vi "Strain Gauge Motion [FPGA Main].vi"() -> ()   [LabVIEW 2017]
doc: "Use this VI to control the cRIO Demo Kit motor and motor drive with a simple set of commands. You can operate the drive in 2 different modes. By default, you can input a velocity setpoint withing +20 or -20 rotations per second and the motor will move to that velocity, limited by the maximum acceleration input. Alternatively, you can turn on the heater mode. This will use the motor like a heater coil within the demo kit by setting the velocity to zero, but enabling full holding current through the drive. You can use the thermocouple in the demo kit to read the temperature of the motor windings. Turn the heating coil on and off by enabling and disabling the drive.\n\nUSING THIS VI: You can run this VI as the top level VI for an easy motion or heater component. Or you can modify this VI to run as a component of a main FPGA application. To do this, replace the front panel objects with target scoped registers, UDVs, or global variables."
uses:
  <vilib>/Platform/TimedLoop/XDataNode/timing_clust.ctl
  <vilib>/Platform/TimedLoop/XDataNode/nitl_modes.ctl
  <vilib>/Platform/TimedLoop/XDataNode/wakeup.ctl
  <vilib>/LabVIEW Targets/FPGA/cRIO/shared/nicrio_ModuleControls/nicrio_cRIO-9503_DriveStatus.ctl
  <vilib>/Motion/MotorControl/_s/nism.stepper.currentScheduler.config.ctl
  <vilib>/Motion/MotorControl/_s/nism.microstepping.rate.ctl
  <vilib>/Motion/MotorControl/_s/nism.pi.gains.sgl.ctl
  <vilib>/Motion/MotorControl/_s/nism.pi.c.currentFeedback.sgl.ctl
  <vilib>/Motion/MotorControl/_s/nism.mdo.antiResonanceData.ctl
  <vilib>/Motion/MotorControl/_s/nism.stepper.currentScheduler.torqueSmoothingCoefficients.ctl
  <vilib>/Motion/MotorControl/_s/nism.pwm.outputs.4phase.ctl
  <vilib>/rvi/DataTransferAndStorage/Container/Common/niFpgaContainerGetUniqueNameForEmu.vi
  <vilib>/rvi/DataTransferAndStorage/Container/Common/niFpgaContainerSetEmuInfo.vi
  <vilib>/rvi/eio/common/nirviEmuReportErrorAndStop.vi
  <vilib>/rvi/Emulation/niFpgaGetClockAttributes.vi
  <vilib>/rvi/Emulation/niFpgaSctlEmulationGetInTimedLoop.vi
  <vilib>/rvi/Emulation/niFpgaEmulationReportErrorSimple.vi
  <vilib>/rvi/eio/common/nirviEmuTemplateMethod_errors.vi
  <vilib>/rvi/Emulation/niFpgaEmulationIsFPGAContextNoSignature.vi
  <vilib>/rvi/Memory/Memory_Emulation/niFpgaMemoryEmulationCacheClearOnFirstRun.vi
  <vilib>/rvi/Memory/Memory_Emulation/nirvimemoryEmulationManagerCache_MakeExclusive.vi
  <vilib>/rvi/Memory/Memory_Emulation/niFpgaMemoryEmulationValidateCache.vi
  <vilib>/rvi/Memory/Memory_Emulation/nirvimemoryEmulationManagerCache_InsertValue.vi
  <vilib>/Utility/error.llb/Clear Errors.vi
  <vilib>/rvi/Memory/Memory_Emulation/nirvimemoryEmulationManagerCache_ReleaseExclusive.vi
  <vilib>/rvi/Memory/Memory_Emulation/nirvimemoryEmulationManagerCache_GetValue.vi
  <vilib>/rvi/Memory/Memory_Emulation/nirvimemoryEmulationManagerCache_SetValue.vi
  <vilib>/rvi/Emulation/niFpgaProcessEmulError.vi
  <vilib>/rvi/Emulation/niFpgaCriticalErrorInLSC.vi
  <vilib>/rvi/occurrence/nirviWaitOnOccurrenceBase.vi
  <vilib>/Motion/MotorControl/_s/nism.rateLimiter.v.fxp.vi
  <vilib>/Motion/MotorControl/_s/nism.stepResolver.fxp.64.32.vi
  <vilib>/Motion/MotorControl/_s/nism.stepper.currentScheduler.advanced.single.vi
  <vilib>/Motion/MotorControl/_s/nism.pi.c.sgl.2phase.2.noAW.vi
  <vilib>/Motion/MotorControl/_s/nism.antiResonance.single.vi
  <vilib>/Motion/MotorControl/_s/nism.9503VoltageTransform.fxp.vi
  <vilib>/rvi/LocalResourceManager/LocalResourceManager.xnode
  <vilib>/eio/EIOMethodNode/EIOMethodNode.xnode
  <vilib>/rvi/DataTransferAndStorage/Container/XNode/niFpgaContainer.xnode
  <vilib>/rvi/DataTransferAndStorage/Register/Emulation/niFpgaRegisterEmulation.vi
  <vilib>/Platform/TimedLoop/XDataNode/XDataNode.xnode
  <vilib>/eio/EIONode/EIONode.xnode
  <vilib>/Motion/MotorControl/NI_SoftMotion_MotorControlIP.lvlib
  <vilib>/Platform/TimedLoop/XDataNode/XDNodeRunTimeDep.lvlib
  <vilib>/Motion/MotorControl/_s/nism.incremental.indexCriteria.ctl
  <vilib>/Motion/MotorControl/_s/nism.encoder.incremental.config.ctl
  <vilib>/Motion/MotorControl/_s/nism.incremental.p.2.vi
panel:
  out "Strain Gauge":sgl
  in  "Heater Mode":bool
  in  "Velocity Setpoint (rev/sec)":sgl caption="velocity setpoint"
  in  "Maximum Acceleration":T1(ring)=enum."High"
  out "Control Loop Timer":u32
  out "Anti-Resonance Enabled?":bool
  out "Pulse Per Revolution":bool
  out "Velocity (rev/sec)":fxp<+/-,32,16> caption="xi" format="%.41g"
  in  "Clear Faults":bool
  in  "Enable Drive":bool
  out "Module Fault Code":u16
  out "Module Fault?":bool
  # "Velocity is limited to +10 or -10 revolutions per second. Positive velocity setpoints equate to counter clockwise rotation.\n\nMax acceleration choices limit the rate of acceleration when changing velocity setpoints.\n\nHeater Mode will stop the motor and always keep full current through the motor windings, generating more heat.\n\nVelocity is the measured encoder velocity and works without the drive enabled. Pulse Per Revolution is the Z encoder pulse and occors exactly once for each revolution."
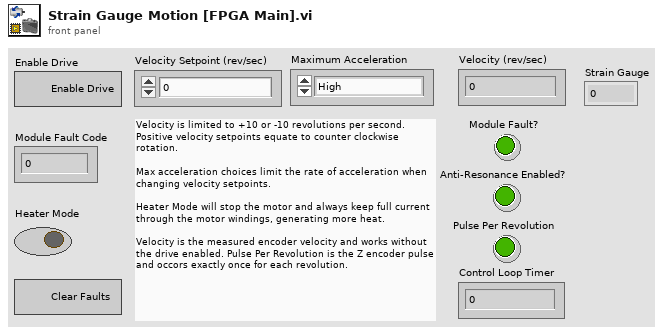
[diagram p1: front panel]
types:
  T1 = enum8{"Extremely Low", "Very Low", "Low", "Medium", "High", "Highest"}
  T2 = typedef "NI_SoftMotion_MotorControlIP.lvlib/nism.encoder.incremental.config.ctl" = cluster{"line a active high?":bool, "line b active high?":bool, "index active high?":bool}
  T3 = typedef "NI_SoftMotion_MotorControlIP.lvlib/nism.incremental.indexCriteria.ctl" = cluster{"a":bool, "b":bool, "z":bool}
  T4 = typedef "XDNodeRunTimeDep.lvlib/timing_clust.ctl" = cluster{"Expected End [f-1]":u64, "Actual End [f-1]":u64, "Finished Late? [f-1]":bool, "Expected End [i-1]":u64, "Actual End [i-1]":u64, "Finished Late? [i-1]":bool, "Expected Start [i]":u64, "Actual Start [i]":u64, "Expected Start [f]":u64, "Actual Start [f]":u64, "Source Name":string, "Structure Name":string, "Period":i64, "Deadline":i64, "Offset":i64, "Start":i64, "Priority":i32, "Timeout":i32, "Mode":T5, "Wakeup Reason":T6, "Error":errorcluster, "Source Type":string, "Secondary Source Type":string, "Global End Time":u64, "Global Start Time":u64, "Frame Duration":u64, "Iteration Duration":u64, "Assigned CPU":i32, "I/O Scan Engine Mode":u32}
  T5 = typedef "XDNodeRunTimeDep.lvlib/nitl_modes.ctl" = enum32{"No Change", "Process missed periods, maintain original phase", "Discard missed periods, maintain original phase", "Process missed periods, ignore original phase", "Discard missed periods, ignore original phase"}
  T6 = typedef "XDNodeRunTimeDep.lvlib/wakeup.ctl" = enum32{"Normal", "Aborted", "Asynchronous wakeup", "Timing source error", "Timed loop error", "Timeout"}
  T7 = typedef "nicrio_cRIO-9503_DriveStatus.ctl" = enum8{"Drive Disabled (Disabled by fault)", "Drive Disabled (Disabled by software)", "Drive Enabled"}
  T8 = typedef "NI_SoftMotion_MotorControlIP.lvlib/nism.pwm.outputs.4phase.ctl" = cluster{"a+":fxp<+/-,16,1>, "a-":fxp<+/-,16,1>, "b+":fxp<+/-,16,1>, "b-":fxp<+/-,16,1>}
  T9 = typedef "NI_SoftMotion_MotorControlIP.lvlib/nism.stepper.currentScheduler.torqueSmoothingCoefficients.ctl" = cluster{"current scheduler : torque smoothing : torque smoothing gain":sgl, "torque smoothing phase":fxp<+/-,16,1>}
  T10 = typedef "NI_SoftMotion_MotorControlIP.lvlib/nism.mdo.antiResonanceData.ctl" = cluster{"coefficient 0":sgl, "coefficient 1":sgl, "coefficient 2":sgl, "coefficient 3":sgl, "coefficient 4":sgl, "coefficient 5":sgl}
  T11 = typedef "NI_SoftMotion_MotorControlIP.lvlib/nism.pi.c.currentFeedback.sgl.ctl" = cluster{"phase a":sgl, "phase b":sgl}
  T12 = typedef "NI_SoftMotion_MotorControlIP.lvlib/nism.pi.gains.sgl.ctl" = cluster{"kp":sgl, "ki":sgl}
  T13 = typedef "NI_SoftMotion_MotorControlIP.lvlib/nism.microstepping.rate.ctl" = enum8{"1 (Full Step)", "2 (Half Step)", "4", "8", "16", "32", "64", "128", "256"}
  T14 = typedef "NI_SoftMotion_MotorControlIP.lvlib/nism.stepper.currentScheduler.config.ctl" = cluster{"rated phase current":sgl, "phase current offset(a)":sgl, "phase current offset(b)":sgl, "reduced current":sgl, "curr. reduction del.":u16}
  T15 = typedef "NI_SoftMotion_MotorControlIP.lvlib/nism.pi.c.currentSetpoint.sgl.ctl" = cluster{"phase a":sgl, "phase b":sgl}
  T16 = typedef "NI_SoftMotion_MotorControlIP.lvlib/nism.pi.c.voltage.sgl.ctl" = cluster{"phase a":sgl, "phase b":sgl}
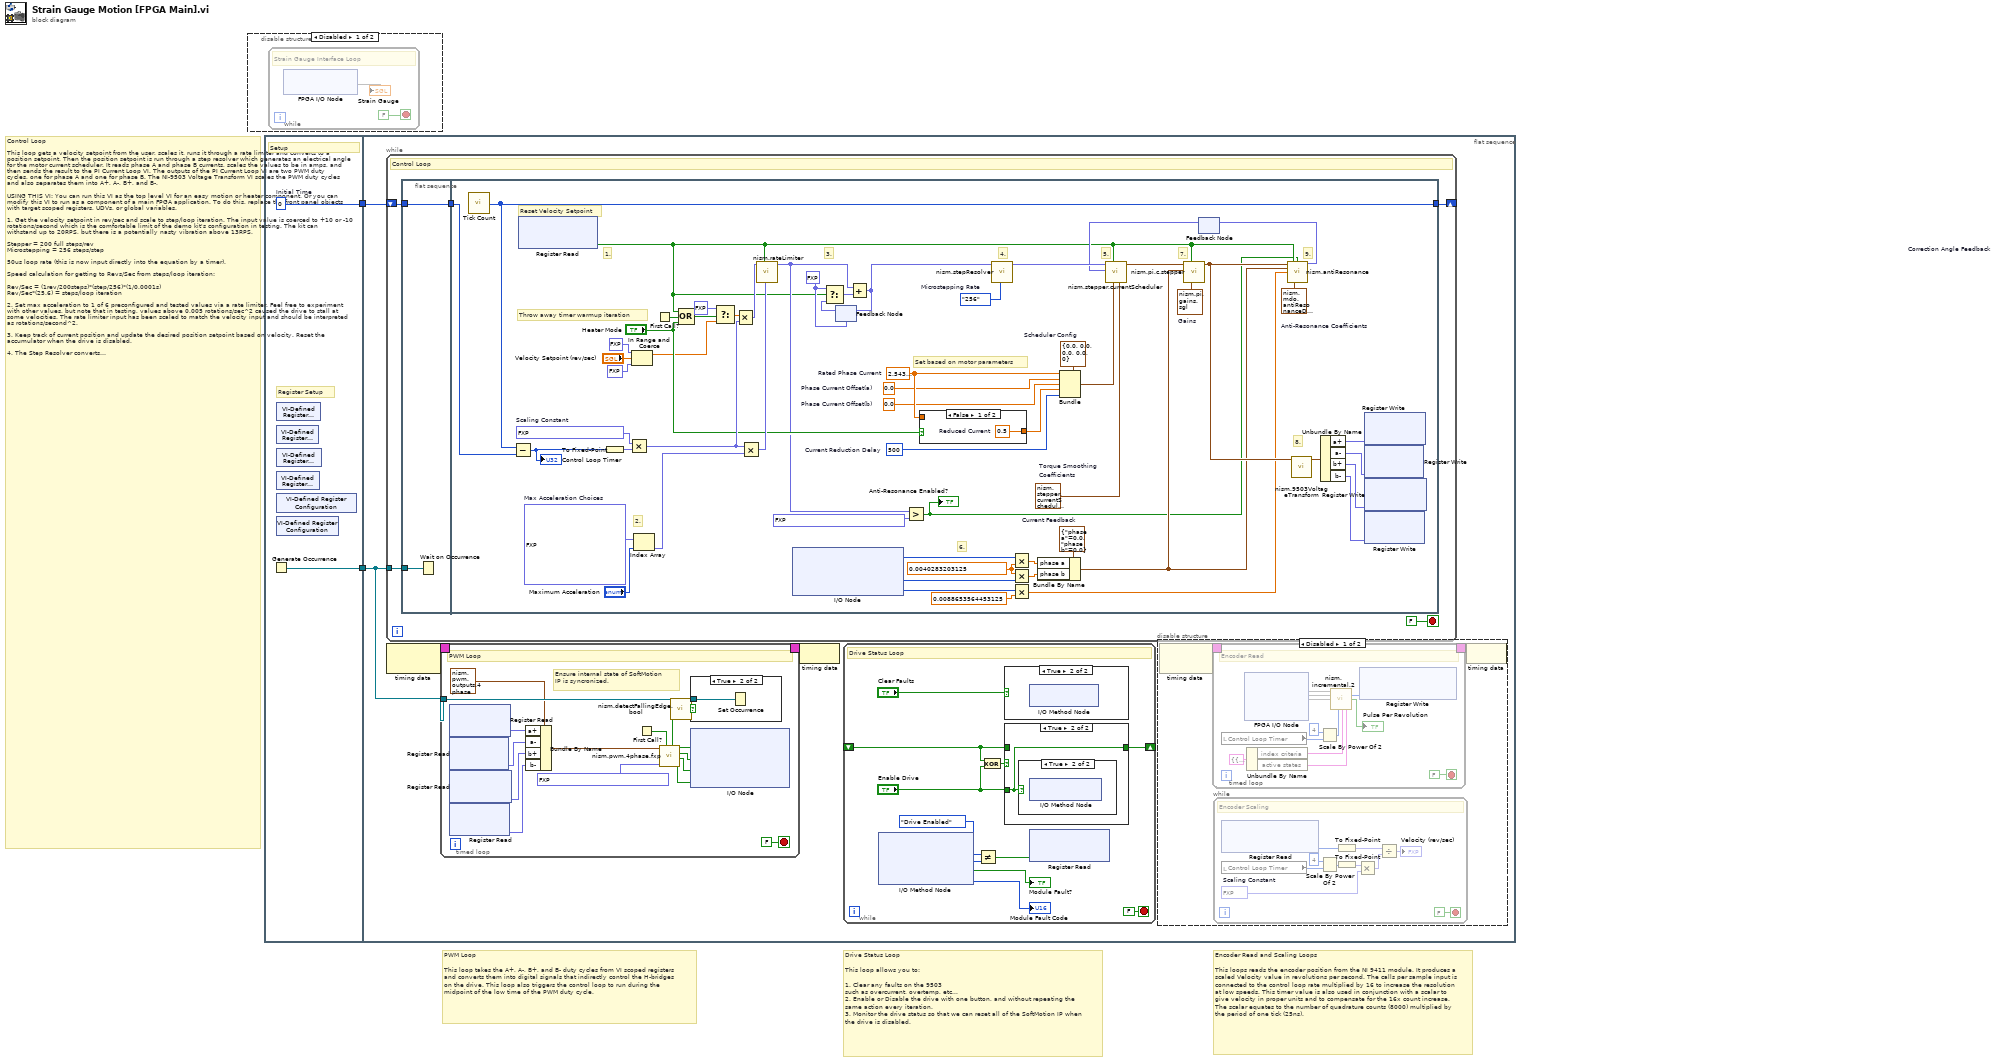
[diagram p0: block diagram]
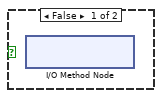
[diagram p6: hidden frame]
diagram:
  # "Encoder Read and Scaling Loops\n\nThis loops reads the encoder position from the NI 9411 module. It produces a scaled Velocity value in revolutions per second. The calls per sample input is connected to the control loop rate multiplied by 16 to increase the resolution at low speeds. This timer value is also used in conjunction with a scalar to give velocity in proper units and to compensate for the 16x count increase. The scalar equates to the number of quadrature counts (8000) multiplied by the period of one tick (25ns)."
  # "Drive Status Loop\n\nThis loop allows you to:\n \n1. Clear any faults on the 9503\nsuch as overcurrent, overtemp, etc...\n2. Enable or Disable the drive with one button, and without repeating the same action every iteration.\n3. Monitor the drive status so that we can reset all of the SoftMotion IP when the drive is disabled."
  # "PWM Loop\n\nThis loop takes the A+, A-, B+, and B- duty cycles from VI scoped registers and converts them into digital signals that indirectly control the H-bridges on the drive. This loop also triggers the control loop to run during the midpoint of the low time of the PWM duty cycle."
  # "Control Loop\n\nThis loop gets a velocity setpoint from the user, scales it, runs it through a rate limiter and converts to a position setpoint. Then the position setpoint is run through a step resolver which generates an electrical angle for the motor current scheduler. It reads phase A and phase B currents, scales the values to be in amps, and then sends the result to the PI Current Loop VI. The outputs of the PI Current Loop VI are two PWM duty cycles, one for phase A and one for phase B. The NI-9503 Voltage Transform VI scales the PWM duty cycles and also separates them into A+, A-, B+, and B-. \n\nUSING THIS VI: You can run this VI as the top level VI for an easy motion or heater component. Or you can modify this VI to run as a component of a main FPGA application. To do this, replace the front panel objects with target scoped registers, UDVs, or global variables.\n\n1. Get the velocity setpoint in rev/sec and scale to step/loop iteration. The input value is coerced to +10 or -10 rotations/second which is the comfortable limit of the demo kit's configuration in testing. The kit can withstand up to 20RPS, but there is a potentially nasty vibration above 13RPS.\n\nStepper = 200 full steps/rev\nMicrostepping = 256 steps/step\n\n50us loop rate (this is now input directly into the equation by a timer).\n\nSpeed calculation for getting to Revs/Sec from steps/loop iteration:\n\nRev/Sec = (1rev/200steps)*(step/256)*(1/0.0001s)\nRev/Sec*(25.6) = steps/loop iteration\n\n2. Set max acceleration to 1 of 6 preconfigured and tested values via a rate limiter. Feel free to experiment with other values, but note that in testing, values above 0.005 rotations/sec^2 caused the drive to stall at some velocities. The rate limiter input has been scaled to match the velocity input and should be interpreted as rotations/second^2. \n\n3. Keep track of current position and update the desired position setpoint based on velocity. Reset the accumulator when the drive is disabled.\n\n4. The Step Resolver converts a position setpoint to an electrical angle between -1 and 1 pi radians.\n\n5. The Motor Current Scheduler converts the electrical angle into phase A and phase B current setpoints. This is also where the rated phase current for the motor and the current reduction settings are implemented. Usually the motor current is reduced by a user-defined amount after a user-defined time period to save power and reduce temperature.  However, to use the motor as a heater for demo purposes with the attached thermocouple, there is an option to keep full current through the motor windings, generating heat. This is called \"heater mode.\" \n\n6. Read the phase A and phase B currents and scale them to be in amps. The current read is triggered by the PWM loop.\n\n7. Run the PI Current Loop to get two PWM duty cycles, one for phase A and one for phase B.  Current control loop gains are calculated based on motor parameters.\n \n8. Scale the PWM duty cycles and split them into four different duty cycles: A+, A-, B+, and B-. Send those duty cycles to the PWM Loop via registers.\n\n9. Applies an anti-resonance algorithm to reduce resonance of the stepper motor allowing for increased speed and performance."
  n1 = disable-structure shown="Disabled" {
    frame Disabled {
      n2 = while {
        stop <- FALSE stop-if-true
        # "Strain Gauge Interface Loop"
        n3 = xnode "FPGA I/O Node"() -> ("Strain Gauge"=→"Strain Gauge")  [unwired: 1 in, 1 out]
      }
    }
    frame Enabled {
    }
  }
  n4 = flat-sequence {
    tunnel: [w6] -> w2
    tunnel: [w5] -> w1
    tunnel: w2 -> [w8]
    tunnel: w1 -> [w7]
    frame #0 {
      w5 = u32 0  # Initial Time
      # "Setup"
      # "Register Setup"
      # "Setup"
      n5 = Generate Occurrence() -> (w6:refnum<k4>)
      n6 = xnode ("VI-Defined Register Configuration")() -> ()  [unwired: 1 out]
      n7 = xnode ("VI-Defined Register Configuration")() -> ()  [unwired: 1 out]
      n8 = xnode ("VI-Defined Register Configuration")() -> ()  [unwired: 1 out]
      n9 = xnode ("VI-Defined Register Configuration")() -> ()  [unwired: 1 out]
      n10 = xnode ("VI-Defined Register Configuration")() -> ()  [unwired: 1 out]
      n11 = xnode ("VI-Defined Register Configuration")() -> ()  [unwired: 1 out]
    }
    frame #1 {
      n12 = while "Control Loop" {
        tunnel: w8 -> [w77]
        shift-right: [w73] -> _
        shift-left: w7 -> [w75]
        stop <- FALSE stop-if-true
        # "Control Loop"
        n13 = flat-sequence {
          tunnel: w77 -> [w79]
          tunnel: [w78] -> w74
          tunnel: w75 -> [w78]
          tunnel: [w138] -> w73
          tunnel: w74 -> [w126]
          frame #0 {
            n14 = Wait on Occurrence(2:w79) -> ()  [unwired: 2 in, 1 out]
          }
          frame #1 {
            w83 = T9 {"current scheduler : torque smoothing : torque smoothing gain"=0.054, "torque smoothing phase"=-0.13800048828125}  # Torque Smoothing Coefficients
            w86 = T10 {"coefficient 0"=0.5555556, "coefficient 1"=0.98511136, "coefficient 2"=0.007444307, "coefficient 3"=1.0, "coefficient 4"=0.9812323, "coefficient 5"=0.009383864}  # Anti-Resonance Coefficients
            w95 = T11 {"phase a"=0.0, "phase b"=0.0}  # Current Feedback
            w96 = T12 {"kp"=1.57, "ki"=0.0235}  # Gains
            w104 = sgl 0.0040283203 ("y")
            w112 = fxp<+/-,32,16>[] [1.52587890625e-05, 4.57763671875e-05, 0.0001068115234375, 0.0005035400390625, 0.001007080078125, 0.0050048828125]  # Max Acceleration Choices
            w118 = fxp<+/-,64,32> 0.0 ("t")
            w125 = fxp<+,16,-9> 0.0012800097465515137  # Scaling Constant
            w93 = nism.microstepping.rate."256"  # Microstepping Rate
            w137 = T14 {"rated phase current"=0.0, "phase current offset(a)"=0.0, "phase current offset(b)"=0.0, "reduced current"=0.0, "curr. reduction del."=0}  # Scheduler Config
            w134 = u16 500  # Current Reduction Delay
            w133 = sgl 0.0  # Phase Current Offset(b)
            w132 = sgl 0.0  # Phase Current Offset(a)
            w136 = sgl 2.544  # Rated Phase Current
            # "9."
            # "Throw away timer warmup iteration"
            # "Reset Velocity Setpoint"
            # "3."
            # "2."
            # "1."
            # "Set based on motor parameters"
            # "5."
            # "4."
            # "6."
            # "8."
            # "7."
            n15 = call "Tick Count"() -> ("Tick Count(Ticks)"=w138:u32)
            n16 = Subtract(x=w138, y=w126) -> (x-y=w98:u32)
            "Control Loop Timer" <- w98
            n17 = xnode ("Register Read")() -> ("Data"=w81:bool)  [unwired: 1 in, 1 out]
            n18 = To Fixed-Point(number=w98) -> (fixed-point=w99:fxp<+,16,16>)  [unwired: 1 in]
            n19 = Multiply(x=w125, y=w99) -> (x*y=w124:fxp<+,32,16>)
            n20 = In Range and Coerce(upper limit=fxp<+/-,32,16> 10.0, x="Velocity Setpoint (rev/sec)", lower limit=fxp<+/-,32,16> -10.0) -> (coerced(x)=w115:sgl)  [unwired: 1 out]
            n21 = Index Array(array=w112, index="Maximum Acceleration") -> (element=w110:fxp<+/-,32,16>)
            n22 = First Call?() -> (First Call?: T/F=w122:bool)
            n23 = Compound Arithmetic op=OR(w81, w122, "Heater Mode") -> (w121:bool)
            n24 = Select(t=fxp<+/-,32,16> 0.0, s=w121, f=w115) -> (s? t:f=w128:sgl)
            n25 = Multiply(x=w128, y=w124) -> (x*y=w130:fxp<+/-,64,32>)
            n26 = Multiply(x=w124, y=w110) -> (x*y=w129:fxp<+/-,64,32>)
            n27 = call-poly <vilib>:"nism.rateLimiter.vi"("max acceleration"=w129, "reset"=w81, "velocity setpoint"=w130) -> ("limited velocity"=w82:fxp<+/-,64,32>)  [unwired: 8 in]
            n28 = xnode "I/O Node"() -> ("Mod1/Phase A Current"=w101:i16, "Mod1/Phase B Current"=w100:i16, "Mod1/Vsup Voltage"=w90:u16)  [unwired: 3 in, 3 out]
            n29 = feedback #1(w118) -> (w119:fxp<+/-,64,32>)
            n30 = Select(t=w118, s=w81, f=w119) -> (s? t:f=w120:fxp<+/-,64,32>)
            n31 = Add(x=w82, y=w120) -> (x+y=w117:fxp<+/-,64,32>)
            n32 = feedback-in #1(w117) -> ()
            n33 = Greater?(x=w82, y=fxp<+/-,64,32> 5.120000000111759) -> (0:w80:bool)
            "Anti-Resonance Enabled?" <- w80
            n34 = case shown="False" "Heater Mode" {
              tunnel: [w139 w140] -> w135
              tunnel: w136 -> [_ w140]
              frame False {
                w139 = sgl 0.5  # Reduced Current
              }
              frame True {
              }
            }
            n35 = call-poly <vilib>:"nism.stepResolver.vi"("microstepping rate"=w93, "position setpoint"=w117) -> ("electrical angle"=w131:fxp<+/-,16,1>)  [unwired: 9 in]
            n36 = Multiply(x=w101, y=w104) -> (x*y=w103:sgl)
            n37 = Multiply(x=w104, y=w100) -> (x*y=w102:sgl)
            n38 = Multiply(x=w90, y=sgl 0.008865356 ("orig 9503")) -> (x*y=w88:sgl)
            n39 = Bundle By Name(cluster=w95, "phase a"=w103, "phase b"=w102) -> (w91:T11)
            n40 = Bundle(cluster=w137, "rated phase current"=w136, "phase current offset(a)"=w132, "phase current offset(b)"=w133, "reduced current"=w135, "curr. reduction del."=w134) -> (w94:T14)
            n41 = feedback #2 "Correction Angle Feedback"() -> (w84:fxp<+/-,16,1>)  [unwired: 1 in]
            n42 = call-poly <vilib>:"nism.stepper.currentScheduler.vi"("torque smoothing coefficients"=w83, "current scheduler config"=w94, "reset"=w81, "correction angle"=w84, "electrical angle"=w131) -> ("current setpoint"=w97:T15)  [unwired: 6 in]
            n43 = call-poly <vilib>:"nism.pi.c.stepper.vi"("gains"=w96, "reset"=w81, "current feedback"=w91, "current setpoint"=w97) -> ("voltage output"=w92:T16)  [unwired: 6 in, 1 out]
            n44 = call-poly <vilib>:"nism.antiResonance.vi"("voltage output"=w92, "reset"=w81, "enable"=w80, "current feedback"=w91, "bus voltage"=w88, "anti-resonance coefficients"=w86) -> ("correction angle"=w85:fxp<+/-,16,1>)  [unwired: 9 in]
            n45 = feedback-in #2(w85) -> ()
            n46 = call-poly <vilib>:"nism.9503VoltageTransform.vi"("voltage output"=w92) -> ("duty cycles"=w109:T8)  [unwired: 10 in]
            n47 = Unbundle By Name(w109) -> ("a+"=w108:fxp<+/-,16,1>, "a-"=w107:fxp<+/-,16,1>, "b+"=w106:fxp<+/-,16,1>, "b-"=w105:fxp<+/-,16,1>)
            n48 = xnode ("Register Write")("Data"=w108) -> ()  [unwired: 1 in, 1 out]
            n49 = xnode ("Register Write")("Data"=w107) -> ()  [unwired: 1 in, 1 out]
            n50 = xnode ("Register Write")("Data"=w106) -> ()  [unwired: 1 in, 1 out]
            n51 = xnode ("Register Write")("Data"=w105) -> ()  [unwired: 1 in, 1 out]
          }
        }
      }
      n52 = node-c288() -> (w10:T4)  [unwired: 1 in]
      n53 = timed-loop "PWM Loop" {
        timing: w10 -> [_]
        timing-out: [_] -> w9
        tunnel: w8 -> [w60]
        stop <- FALSE stop-if-true
        # "Ensure internal state of SoftMotion\nIP is syncronized."
        # "PWM Loop"
        n54 = xnode ("Register Read")() -> ("Data"=w57:fxp<+/-,16,1>)  [unwired: 1 in, 1 out]
        n55 = xnode ("Register Read")() -> ("Data"=w56:fxp<+/-,16,1>)  [unwired: 1 in, 1 out]
        n56 = xnode ("Register Read")() -> ("Data"=w55:fxp<+/-,16,1>)  [unwired: 1 in, 1 out]
        n57 = xnode ("Register Read")() -> ("Data"=w54:fxp<+/-,16,1>)  [unwired: 1 in, 1 out]
        n58 = Bundle By Name(cluster=T8 {"a+"=0.0, "a-"=0.0, "b+"=0.0, "b-"=0.0} ("duty cycles"), "a+"=w57, "a-"=w56, "b+"=w55, "b-"=w54) -> (w58:T8)
        n59 = First Call?() -> (First Call?: T/F=w52:bool)
        n60 = call <vilib>:"nism.pwm.4phase.fxp.vi"("reset"=w52, "frequency"=fxp<+,32,0> 0.0005000000819563866, "duty cycles"=w58) -> ("phase b-"=w63:bool, "phase b+"=w64:bool, "phase a-"=w65:bool, "phase a+"=w66:bool, "trigger"=w62:bool)  [unwired: 4 in]
        n61 = call <vilib>:"nism.detectFallingEdge.bool.vi"("x"=w62) -> ("y"=w61:bool)
        n62 = case shown="True" w61 {
          tunnel: w60 -> [_ w68]
          frame False {
          }
          frame True {
            n63 = Set Occurrence(w68) -> ()
          }
        }
        n64 = xnode "I/O Node"("Mod1/Phase A Pos"=w66, "Mod1/Phase A Neg"=w65, "Mod1/Phase B Pos"=w64, "Mod1/Phase B Neg"=w63) -> ()  [unwired: 4 in, 4 out]
      }
      n65 = node-c288(w9) -> ()
      n66 = while "Drive Status Loop" {
        shift-right: [w47] -> _
        shift-left: _ -> [w46]
        stop <- FALSE stop-if-true
        # "Drive Status Loop"
        n67 = xnode "I/O Method Node"() -> ("Drive Status"=w43:T7, "Module Fault?"=→"Module Fault?":bool, "Module Fault Code"=→"Module Fault Code":u16)  [unwired: 1 in, 1 out]
        n68 = Not Equal?(x=nicrio_cRIO-9503_DriveStatus."Drive Enabled" ("y"), y=w43) -> (x != y?=w41:bool)
        n69 = Exclusive Or(1:"Enable Drive", 2:w46) -> (0:w48:bool)
        n70 = case shown="True" "Clear Faults" {
          frame False {
          }
          frame True {
            n71 = xnode "I/O Method Node"() -> ()  [unwired: 1 in, 1 out]
          }
        }
        n72 = case shown="True" w48 {
          tunnel: "Enable Drive" -> [_ w51]
          tunnel: [w50 w51] -> w47
          tunnel: w46 -> [w50 _]
          frame False {
          }
          frame True {
            n73 = case shown="True" w51 {
              frame False {
                n74 = xnode "I/O Method Node"() -> ()  [unwired: 1 in, 1 out]
              }
              frame True {
                n75 = xnode "I/O Method Node"() -> ()  [unwired: 1 in, 1 out]
              }
            }
          }
        }
        n76 = xnode ("Register Read")("Data"=w41) -> ()  [unwired: 1 in, 1 out]
      }
      n77 = disable-structure shown="Disabled" {
        frame Disabled {
          n78 = node-c288() -> (w12:T4)  [unwired: 1 in]
          n79 = timed-loop "Encoder Read" {
            timing: w12 -> [_]
            timing-out: [_] -> w11
            stop <- FALSE stop-if-true
            # "Encoder Read"
            n80 = local read "Control Loop Timer"() -> (w25:u32)
            n81 = xnode "FPGA I/O Node"() -> ("EncoderA"=w29, "EncoderB"=w28, "EncoderZ"=w27)  [unwired: 3 in, 3 out]
            n82 = Unbundle By Name(cluster{"active states":T2, "index criteria":T3} {"active states"={"line a active high?"=TRUE, "line b active high?"=TRUE, "index active high?"=TRUE}, "index criteria"={"a"=FALSE, "b"=FALSE, "z"=TRUE}} ("Encoder Config")) -> ("index criteria"=w33:T3, "active states"=w32:T2)
            n83 = Scale By Power Of 2(n=i16 4, x=w25) -> (x*2^n=w24:u32)
            n84 = call-poly <vilib>:"nism.incremental.2.vi"("a phase"=w29, "b phase"=w28, "z phase"=w27, "calls per sample"=w24, "index criteria"=w33, "active states"=w32) -> ("velocity"=w26:i16, "index"=→"Pulse Per Revolution":bool)  [unwired: 6 in, 2 out]
            n85 = xnode ("Register Write")("Data"=w26) -> ()  [unwired: 1 in, 1 out]
          }
          n86 = while "Encoder Scaling" {
            stop <- FALSE stop-if-true
            w20 = fxp<+,8,-12> 0.0002002716064453125  # Scaling Constant
            # "Encoder Scaling"
            n87 = local read "Control Loop Timer"() -> (w16:u32)
            n88 = xnode ("Register Read")() -> ("Data"=w18:i16)  [unwired: 1 in, 1 out]
            n89 = Scale By Power Of 2(n=i16 4, x=w16) -> (x*2^n=w14:u32)
            n90 = To Fixed-Point(number=w18) -> (fixed-point=w17:fxp<+/-,32,16>)  [unwired: 1 in]
            n91 = To Fixed-Point(number=w14) -> (fixed-point=w13:fxp<+,16,16>)  [unwired: 1 in]
            n92 = Multiply(x=w13, y=w20) -> (x*y=w22:fxp<+/-,32,16>)
            n93 = Divide(x=w17, y=w22) -> (x/y=→"Velocity (rev/sec)":fxp<+/-,32,16>)
          }
          n94 = node-c288(w11) -> ()
        }
        frame Enabled {
        }
      }
    }
  }
